vi "Read Display_LE.vi"(0 "LEUI_LEDs_Actual":T1, 1 "LEUI_LEDs_Expected":T1, 2 "Care":T1, 11 "Error In":errorcluster) -> (4 "Pass/Fail?":bool, 6 "Report Text":string, 8 "Binary Number Displayed":u32, 15 "Error Out":errorcluster)   [LabVIEW 2016, in "TLMB.lvlib"]
uses:
  Projects/TLMB.lvlib
  controls/LEUI_LEDs.ctl
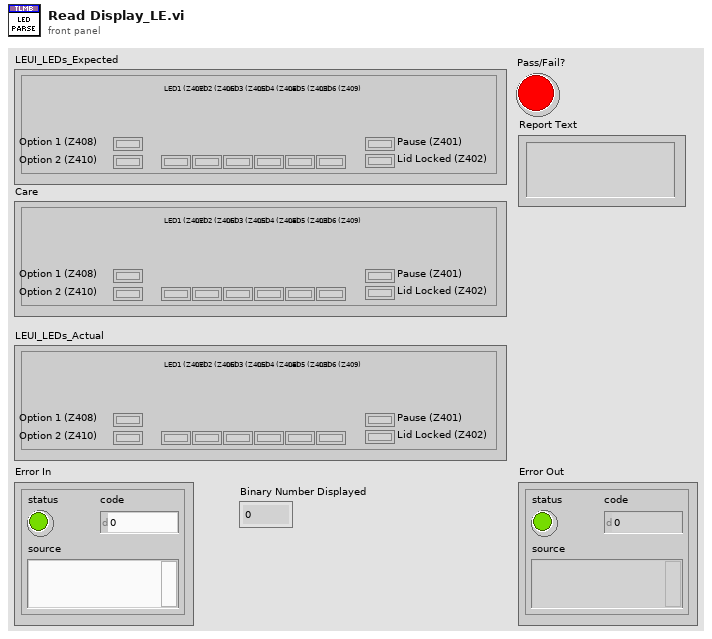
[diagram p1: front panel]
types:
  T1 = typedef "TLMB.lvlib/LEUI_LEDs.ctl" = cluster{"Pause (Z401)":bool, "Lid Locked (Z402)":bool, "LED1 (Z407)":bool, "LED2 (Z406)":bool, "LED3 (Z405)":bool, "LED4 (Z404)":bool, "LED5 (Z403)":bool, "LED6 (Z409)":bool, "Option 1 (Z408)":bool, "Option 2 (Z410)":bool}
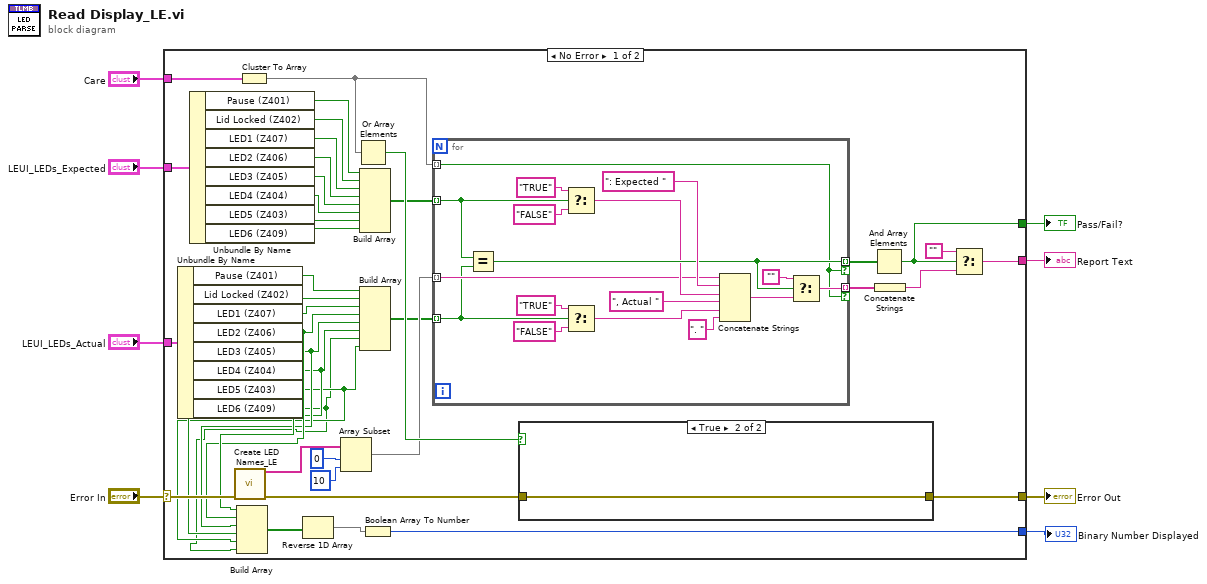
[diagram p0: block diagram]
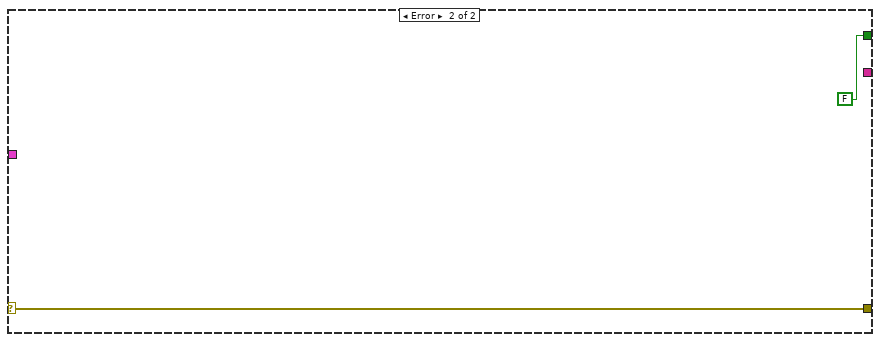
[diagram p3: hidden frame]
diagram:
  n1 = case shown="No Error" "Error In" {
    selector: "Error In" -> [w45 w68]
    tunnel: [w29 w68] -> w6
    tunnel: [w46 _] -> w8
    tunnel: "Care" -> [w43 _]
    tunnel: "LEUI_LEDs_Expected" -> [w19 _]
    tunnel: "LEUI_LEDs_Actual" -> [w22 _]
    tunnel: [w20 FALSE] -> w7
    tunnel: [w9 _] -> w1
    frame No Error {
      n2 = Unbundle By Name(w22) -> ("Pause (Z401)"=w24:bool, "Lid Locked (Z402)"=w23:bool, "LED1 (Z407)"=w15:bool, "LED2 (Z406)"=w14:bool, "LED3 (Z405)"=w13:bool, "LED4 (Z404)"=w12:bool, "LED5 (Z403)"=w11:bool, "LED6 (Z409)"=w10:bool)
      n3 = Unbundle By Name(w19) -> ("Pause (Z401)"=w33:bool, "Lid Locked (Z402)"=w32:bool, "LED1 (Z407)"=w31:bool, "LED2 (Z406)"=w30:bool, "LED3 (Z405)"=w28:bool, "LED4 (Z404)"=w27:bool, "LED5 (Z403)"=w26:bool, "LED6 (Z409)"=w25:bool)
      n4 = call "Create LED Names_LE.vi"("Error In"=w45) -> ("Names"=w37:string[], "Error Out"=w42:errorcluster)  [unwired: 13 in]
      n5 = Build Array(w15, w14, w13, w12, w11, w10) -> (w17:bool[])
      n6 = Cluster To Array(cluster=w43) -> (array=w18:bool[])
      n7 = Reverse 1D Array(array=w17) -> (reversed array=w16:bool[])
      n8 = Array Subset(array=w37, index=0, length=10) -> (w38:string[])
      n9 = Or Array Elements(Boolean array=w18) -> (logical OR=w44:bool)
      n10 = Build Array(w33, w32, w31, w30, w28, w27, w26, w25) -> (w41:bool[])
      n11 = Build Array(w24, w23, w15, w14, w13, w12, w10, w11) -> (w21:bool[])
      n12 = Boolean Array To Number(Boolean array=w16) -> (number=w9:u32)
      n13 = for {
        tunnel: w21 -> [w48] mode=indexing
        tunnel: w41 -> [w49] mode=indexing
        tunnel: [w59] -> w36 mode=indexing if=w57
        tunnel: [w58] -> w34 mode=indexing if=w57
        tunnel: w18 -> [w57] mode=indexing
        tunnel: w38 -> [w50] mode=indexing
        n14 = Equal?(x=w49, y=w48) -> (x = y?=w58:bool)
        n15 = Select(t="TRUE" ("string"), s=w49, f="FALSE" ("string")) -> (s? t:f=w51:string)
        n16 = Select(t="TRUE" ("string"), s=w48, f="FALSE" ("string")) -> (s? t:f=w54:string)
        n17 = Concatenate Strings(w50, ": Expected " ("string"), w51, ", Actual " ("string"), w54, ". " ("string")) -> (w60:string)
        n18 = Select(t="", s=w58, f=w60) -> (s? t:f=w59:string)
      }
      n19 = case shown="True" w44 {
        tunnel: w42 -> [w65 w66]
        tunnel: [w65 w66] -> w29
        frame False {
        }
        frame True {
        }
      }
      n20 = And Array Elements(Boolean array=w34) -> (logical AND=w20:bool)
      n21 = Concatenate Strings(w36) -> (w35:string)
      n22 = Select(t="", s=w20, f=w35) -> (s? t:f=w46:string)
    }
    frame Error {
    }
  }
  "Report Text" <- w8
  "Pass/Fail?" <- w7
  "Error Out" <- w6
  "Binary Number Displayed" <- w1
